vi "Create RPC Client Method.vi"(8 "error in (no error)":errorcluster, 10 "RPC Method Parameters":T1, 11 "Server class in":refnum<vi>) -> (0 "error out":errorcluster, 2 "Newly created ?":bool, 3 "Server class out":refnum<vi>)   [LabVIEW 2019, in "gRPC Scripting Tools.lvlib"]
uses:
  gRPC Scripting Tools.lvlib
  TypeDefs/RPC Method Parameters.ctl
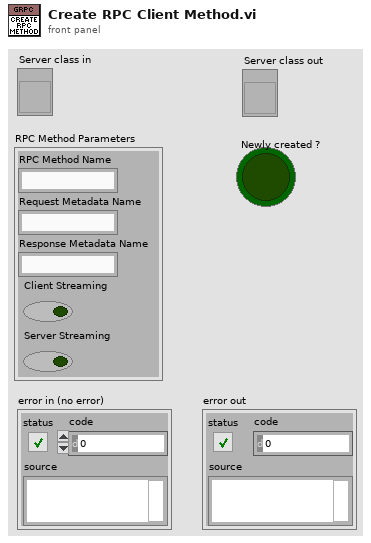
[diagram p1: front panel]
types:
  T1 = typedef "gRPC Scripting Tools.lvlib/RPC Method Parameters.ctl" = cluster{"RPC Method Name":string, "Request Metadata Name":string, "Response Metadata Name":string, "Client Streaming":bool, "Server Streaming":bool}
  T2 = enum32{"invalid VI type", "Standard VI", "Control VI", "Global VI", "Polymorphic VI", "Configuration VI", "SubSystem", "Facade VI", "Method VI"}
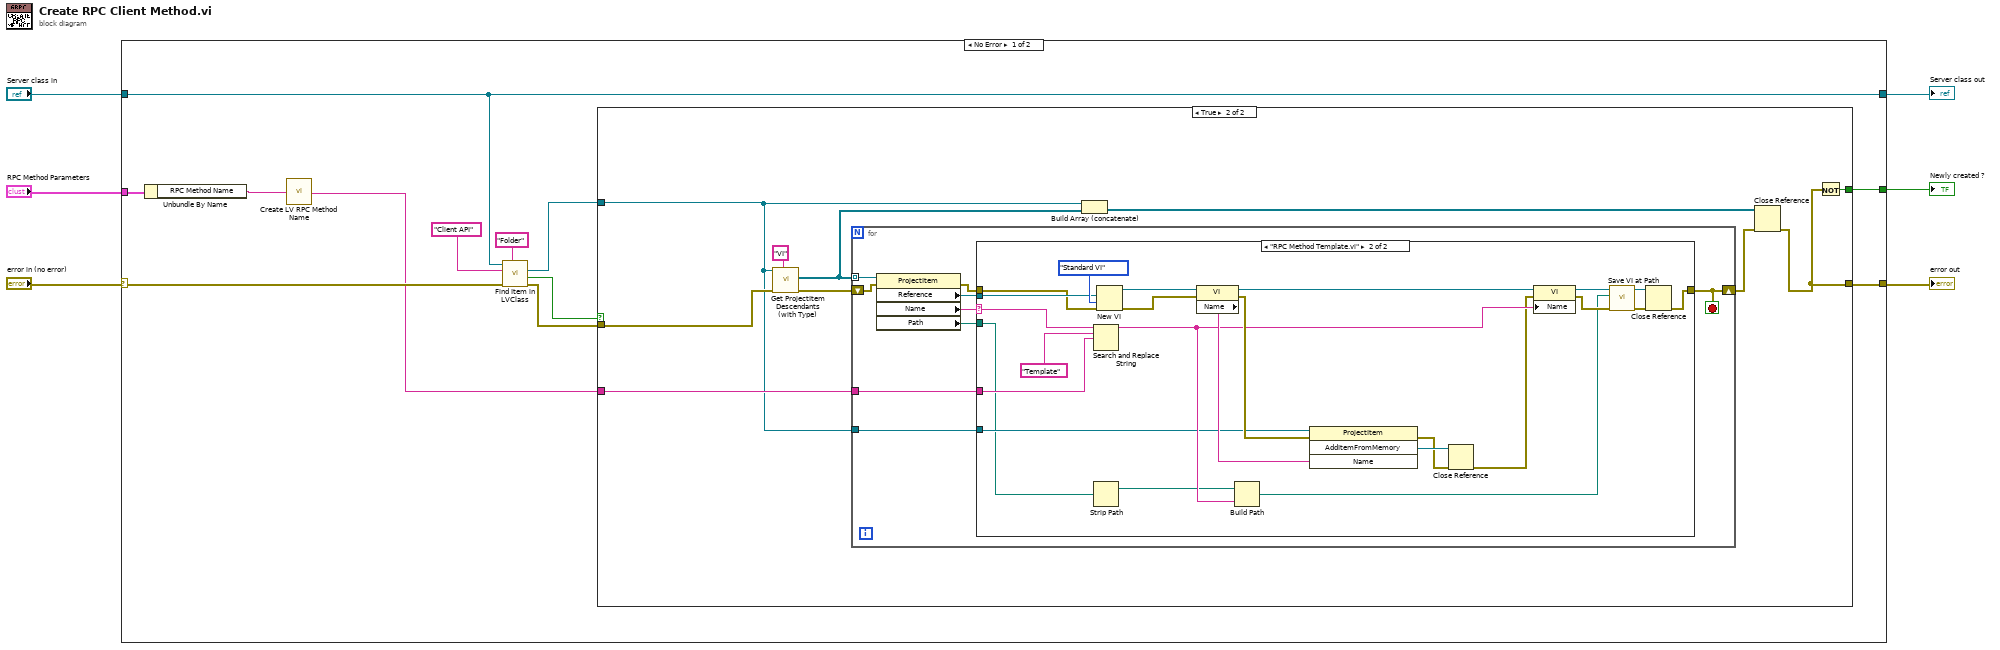
[diagram p0: block diagram]
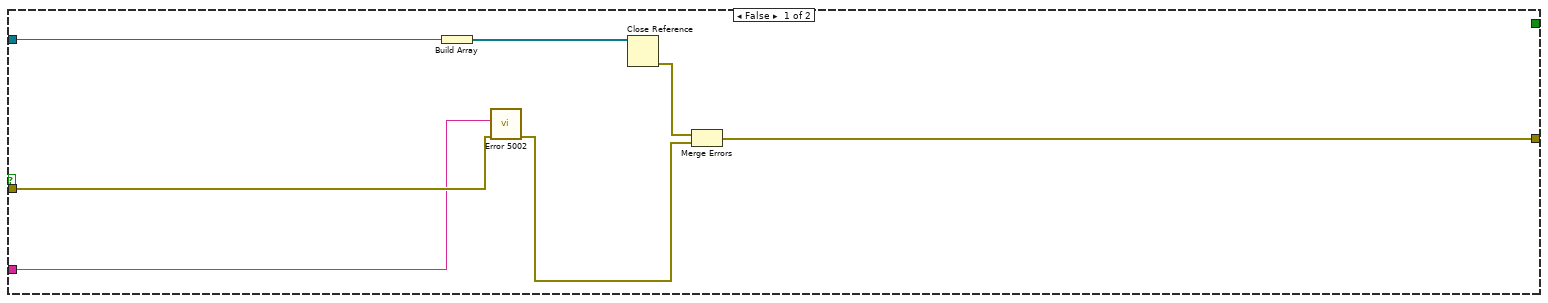
[diagram p2: hidden frame]
diagram:
  n1 = case shown="No Error" "error in (no error)" {
    selector: "error in (no error)" -> [w14 w71]
    tunnel: "Server class in" -> [w13 w70]
    tunnel: [w16 w71] -> w5
    tunnel: [w13 w70] -> w3
    tunnel: [w12 _] -> w2
    tunnel: "RPC Method Parameters" -> [w11 _]
    frame No Error {
      n2 = Unbundle By Name(w11) -> ("RPC Method Name"=w10:string)
      n3 = call "Create LV RPC Method Name.vi"("Proto Parser RPC Method Name in"=w10) -> ("LV RPC Method Name out"=w9:string)
      n4 = call "Find Item in LVClass.vi"("Item Type"="Folder", "error in (no error)"=w14, "Item Name"="Client API", "Class Item in"=w13) -> ("error out"=w7:errorcluster, "Found?"=w8:bool, "Project Item (Class Item)"=w15:refnum<vi>)  [unwired: 4 in, 1 out]
      n5 = case shown="True" w8 {
        tunnel: w15 -> [w24 w26]
        tunnel: w7 -> [w25 w27]
        tunnel: [w19 w34] -> w16
        tunnel: w9 -> [w23 w35]
        tunnel: [_ w33] -> w12
        frame False {
          n6 = Build Array(w24) -> (w22:refnum<vi>[])
          n7 = call "Error 5002.vi"("error in (no error)"=w25, "Method Name"=w23) -> ("error out"=w21:errorcluster)  [unwired: 9 in]
          n8 = Close Reference(reference=w22) -> (error out=w20:errorcluster)  [unwired: 1 in]
          n9 = Merge Errors(w20, w21) -> (w19:errorcluster)
        }
        frame True {
          n10 = call "Get ProjectItem Descendants (with Type).vi"("Type"="VI", "error in (no error)"=w27, "ProjectItem in"=w26) -> ("error out"=w29:errorcluster, "All Descendents"=w30:refnum<vi>[])  [unwired: 6 in, 1 out]
          n11 = for {
            tunnel: w30 -> [w44] mode=indexing
            tunnel: w26 -> [w38]
            tunnel: w35 -> [w39]
            shift-right: [w36] -> w28
            shift-left: w29 -> [w43]
            stop <- w36 stop-if-true
            n12 = property class="ProjectItem"(reference=w44, error in=w43) -> (error out=w37:errorcluster, "Reference"=w41:refnum<vi>, "Name"=w42:string, "Path"=w40:path)  [unwired: 1 out]
            n13 = case shown="\"RPC Method Template.vi\"" w42 {
              selector: w42 -> [_ w52]
              tunnel: w41 -> [_ w53]
              tunnel: w40 -> [_ w47]
              tunnel: w39 -> [_ w48]
              tunnel: w38 -> [_ w51]
              tunnel: w37 -> [w45 w50]
              tunnel: [w45 w49] -> w36
              frame "None", Default {
              }
              frame "RPC Method Template.vi" {
                n14 = Search and Replace String(input string=w52, search string="Template", replace string=w48) -> (result string=w60:string)  [unwired: 5 in, 3 out]
                n15 = Strip Path(path=w47) -> (stripped path=w46:path)  [unwired: 1 out]
                n16 = New VI(8:w50, 9:T2."Standard VI" ("vi type (standard vi)"), 10:w53) -> (0:w64:errorcluster, 3:w67:refnum<vi>)  [unwired: 1 in, 3 out]
                n17 = property class="VI"(reference=w67, error in=w64) -> (reference out=w65:refnum<vi>, error out=w63:errorcluster, "Name"=w68:string)
                n18 = Build Path(base path=w46, name or relative path=w60) -> (appended path=w59:path)
                n19 = invoke class="ProjectItem" method="AddItemFromMemory"(reference=w51, error in=w63, "Name"=w68) -> (error out=w55:errorcluster, "AddItemFromMemory"=w56:refnum<vi>)  [unwired: 1 in, 2 out]
                n20 = Close Reference(reference=w56, error in (no error)=w55) -> (error out=w54:errorcluster)
                n21 = property class="VI"(reference=w65, error in=w54, "Name"=w60) -> (reference out=w62:refnum<vi>, error out=w61:errorcluster)
                n22 = call "Save VI at Path.vi"("error in (no error)"=w61, "Path"=w59, "VI in"=w62) -> ("error out"=w58:errorcluster, "VI out"=w57:refnum<vi>)  [unwired: 6 in, 1 out]
                n23 = Close Reference(reference=w57, error in (no error)=w58) -> (error out=w49:errorcluster)
              }
            }
          }
          n24 = Build Array (concatenate)(w26, w30) -> (w32:refnum<vi>[])
          n25 = Close Reference(reference=w32, error in (no error)=w28) -> (error out=w34:errorcluster)
          n26 = Not(x=w34) -> (.not. x?=w33:bool)
        }
      }
    }
    frame Error {
    }
  }
  "error out" <- w5
  "Server class out" <- w3
  "Newly created ?" <- w2
